vi "ep_Difference Operation.vi"(7 "reset? (F)":bool, 8 "error in (no error)":errorcluster, 9 "previous value":dbl format="%#_13g", 11 "signal in":dbl[](array[numeric])) -> (0 "error out":errorcluster, 1 "next  value":dbl format="%#_13g", 3 "signal out":dbl[](array[numeric]))   [LabVIEW 2014, in "NI_EP_Motor Monitoring.lvlib"]
uses:
  <vilib>/addons/Electrical Power/Motor Monitoring/NI_EP_Motor Monitoring.lvlib
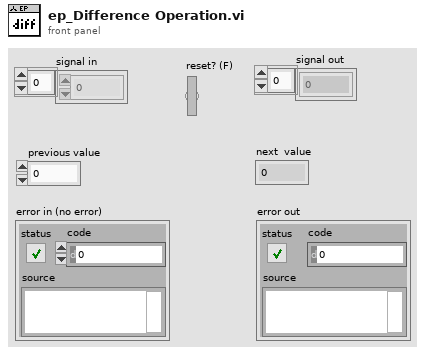
[diagram p1: front panel]
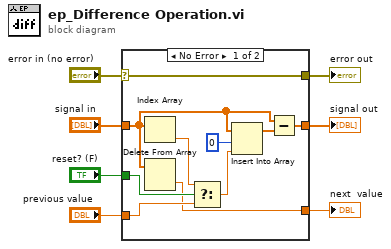
[diagram p0: block diagram]
diagram:
  n1 = case shown="No Error" "error in (no error)" {
    selector: "error in (no error)" -> [w16 w18]
    tunnel: [w16 w18] -> w6
    tunnel: "reset? (F)" -> [w17 _]
    tunnel: "previous value" -> [w13 _]
    tunnel: "signal in" -> [w15 _]
    tunnel: [w12 _] -> w2
    tunnel: [w14 _] -> w1
    frame No Error {
      n2 = Index Array(array=w15) -> (element=w8:dbl)  [unwired: 1 in]
      n3 = Delete From Array(array=w15) -> (deleted portion=w12:dbl)  [unwired: 2 in, 1 out]
      n4 = Select(t=w8, s=w17, f=w13) -> (s? t:f=w9:dbl)
      n5 = Insert Into Array(array=w15, index=0, new element=w9) -> (w11:dbl[])
      n6 = Subtract(x=w15, y=w11) -> (x-y=w14:dbl[])
    }
    frame Error {
    }
  }
  "error out" <- w6
  "next  value" <- w2
  "signal out" <- w1
